vi "UDP Data Link - Action VIs - ActionVIOnDelete.vi"(6 "All deleted Refs":T1[](array[typedef]) format="%.0x", 8 "error in (no error)":errorcluster, 11 "Item Ref in":T1 format="%.0x") -> (0 "error out":errorcluster, 3 "Item Ref out":T1 format="%.0x")   [LabVIEW 2012, in "UDP Data Link System Explorer.lvlib"]
uses:
  UDP Data Link System Explorer.lvlib
  <vilib>/NI Veristand/Custom Device API/Custom Device Item Ref.ctl
  Shared/UDP Data Link Global.vi
  <vilib>/NI Veristand/Custom Device Tools/Custom Device Utility Library/NI VeriStand - Search for Item by GUID.vi
  <vilib>/NI Veristand/Custom Device Tools/Custom Device Utility Library/Custom Device Utility Library.lvlib
  Shared/UDP Data Link Shared.lvlib
  <vilib>/NI Veristand/Custom Device API/Custom Device API.lvlib
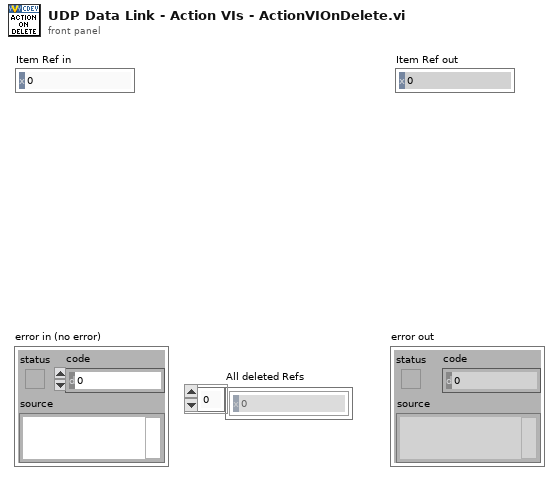
[diagram p1: front panel]
types:
  T1 = typedef "Custom Device API.lvlib/Custom Device Item Ref.ctl" = u64
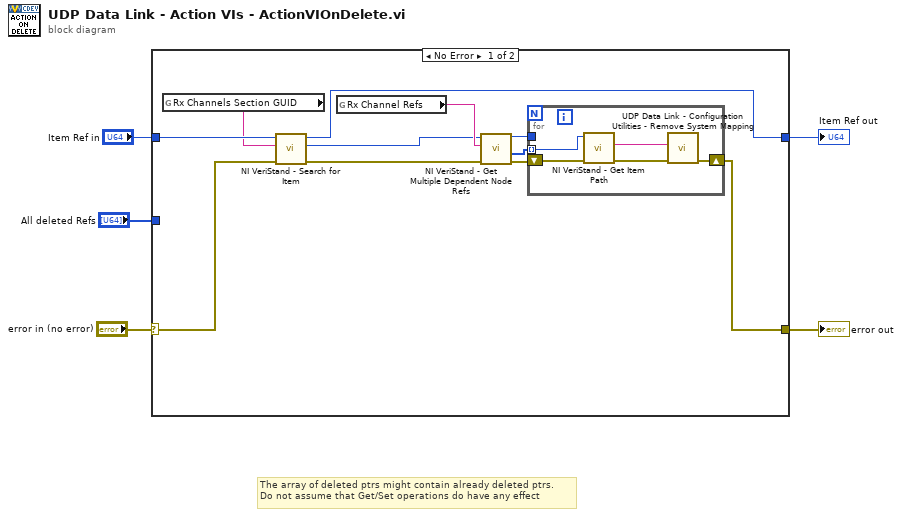
[diagram p0: block diagram]
diagram:
  # "The array of deleted ptrs might contain already deleted ptrs.\nDo not assume that Get/Set operations do have any effect"
  n1 = case shown="No Error" "error in (no error)" {
    selector: "error in (no error)" -> [w14 w23]
    tunnel: [w10 w23] -> w4
    tunnel: "Item Ref in" -> [w16 w22]
    tunnel: [w6 w22] -> w2
    tunnel: "All deleted Refs" -> [_ _]
    frame No Error {
      n2 = global read "UDP Data Link Global.vi" "Rx Channels Section GUID"() -> (w15:string)
      n3 = call-poly <vilib>:"NI VeriStand - Search for Item.vi"("error in"=w14, "Item GUID"=w15, "Section Ref in"=w16) -> ("error out"=w13:errorcluster, "Item Ref"=w7:T1, "Section Ref out"=w6:T1)  [unwired: 5 in, 1 out]
      n4 = global read "UDP Data Link Global.vi" "Rx Channel Refs"() -> (w12:string)
      n5 = call <vilib>:"NI VeriStand - Get Multiple Dependent Node Refs.vi"("error in (no error)"=w13, "Base Property Name"=w12, "Item Ref in"=w7) -> ("error out"=w11:errorcluster, "Dependent Node Refs"=w8:T1[], "Item Ref out"=w9:T1)  [unwired: 6 in]
      n6 = for {
        shift-right: [w21] -> w10
        shift-left: w11 -> [w20]
        tunnel: w9 -> [_]
        tunnel: w8 -> [w19] mode=indexing
        n7 = call <vilib>:"NI VeriStand - Get Item Path.vi"("error in (no error)"=w20, "Item Ref in"=w19) -> ("error out"=w17:errorcluster, "Path"=w18:string)  [unwired: 6 in, 2 out]
        n8 = call "UDP Data Link - Configuration Utilities - Remove System Mapping.vi"("error in (no error)"=w17, "Channel Path Destination"=w18) -> ("error out"=w21:errorcluster)  [unwired: 8 in, 1 out]
      }
    }
    frame Error {
    }
  }
  "error out" <- w4
  "Item Ref out" <- w2
